vi "HalfAdder.vi"() -> ()   [LabVIEW 2015]
panel:
  out "S":bool
  in  "input 2":bool
  in  "input 1":bool
  out "C":bool
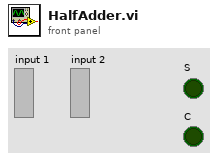
[diagram p1: front panel]
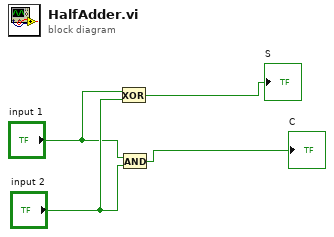
[diagram p0: block diagram]
diagram:
  n1 = Exclusive Or(1:"input 2", 2:"input 1") -> (0:→"S":bool)
  n2 = And(x="input 1", y="input 2") -> (x .and. y?=→"C":bool)
